vi "Write Signal Generator 2.lvclass.vi"(10 "Signal Generator.lvclass":refnum<class "Signal Generator.lvclass">, 11 "IMD in":refnum<class "IMD.lvclass">) -> (3 "IMD out":refnum<class "IMD.lvclass">)   [LabVIEW 2020, in "IMD.lvclass"]
uses:
  IMD.lvclass
  Instruments/Signal Generator/Signal Generator.lvclass
  IMD.lvclass/IMD.ctl
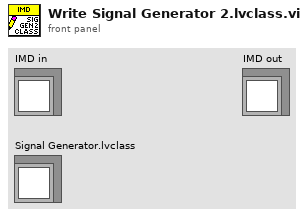
[diagram p1: front panel]
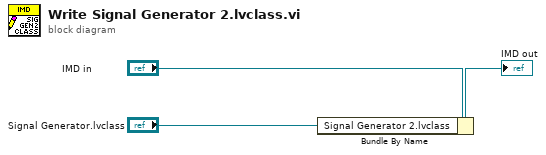
[diagram p0: block diagram]
diagram:
  n1 = Bundle By Name(cluster="IMD in", "Signal Generator 2.lvclass"="Signal Generator.lvclass") -> (→"IMD out":refnum<class "IMD.lvclass">)
